vi "Get Dependencies.vi"(0 "VI path":path, 11 "error in (no error)":errorcluster) -> (4 "Existing dependencies":path[](array[path]), 15 "error out":errorcluster)   [LabVIEW 2021, in "Multiple Migrator.lvlib"]
uses:
  Multiple Migrator.lvlib
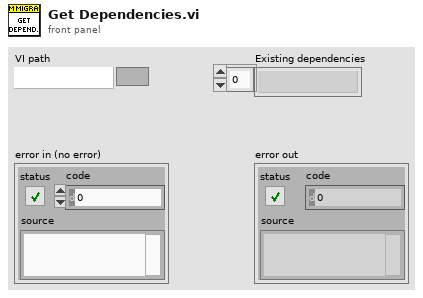
[diagram p1: front panel]
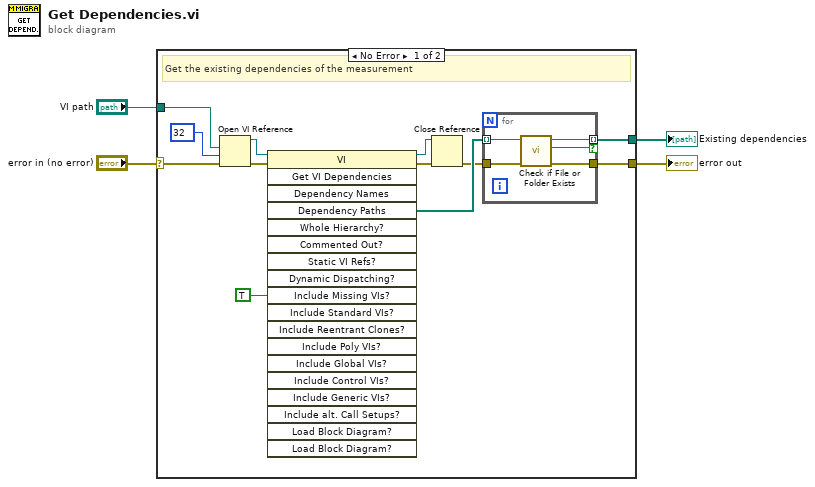
[diagram p0: block diagram]
diagram:
  n1 = case shown="No Error" "error in (no error)" {
    selector: "error in (no error)" -> [w5 _]
    tunnel: [w16 _] -> w4
    tunnel: [w15 _] -> w3
    tunnel: "VI path" -> [w7 _]
    frame No Error {
      # "Get the existing dependencies of the measurement"
      n2 = Open VI Reference(vi path=w7, options=32, error in (no error)=w5) -> (vi reference=w8:refnum<vi>, error out=w9:errorcluster)  [unwired: 3 in]
      n3 = invoke class="VI" method="Get VI Dependencies"(reference=w8, error in=w9, "Include Missing VIs?"=TRUE ("Include Missing Items?")) -> (reference out=w11:refnum<vi>, error out=w10:errorcluster, "Dependency Paths"=w14:path[])  [unwired: 16 in, 16 out]
      n4 = Close Reference(reference=w11, error in (no error)=w10) -> (error out=w13:errorcluster)
      n5 = for {
        tunnel: w13 -> [w21]
        tunnel: w14 -> [w20] mode=indexing
        tunnel: [w19] -> w16 mode=indexing if=w18
        tunnel: [w17] -> w15
        n6 = call <vilib>:"Check if File or Folder Exists.vi"("error in (no error)"=w21, "path"=w20) -> ("error out"=w17:errorcluster, "file or folder exists?"=w18:bool, "dup path"=w19:path)  [unwired: 7 in]
      }
    }
    frame Error {
    }
  }
  "Existing dependencies" <- w4
  "error out" <- w3
